vi "Dialog-Super Password.vi"(8 "error in":errorcluster, 11 "Please Enter the Developer Password":string) -> (0 "error out":errorcluster, 2 "Password Out":string, 3 "Cancelled?":bool)   [LabVIEW 2018]
doc: "Use this template to create a dialog box with event handling."
panel:
  in  "Yes":bool
  in  "Cancel":bool
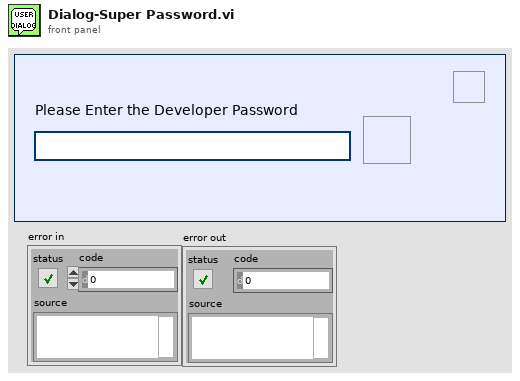
[diagram p1: front panel]
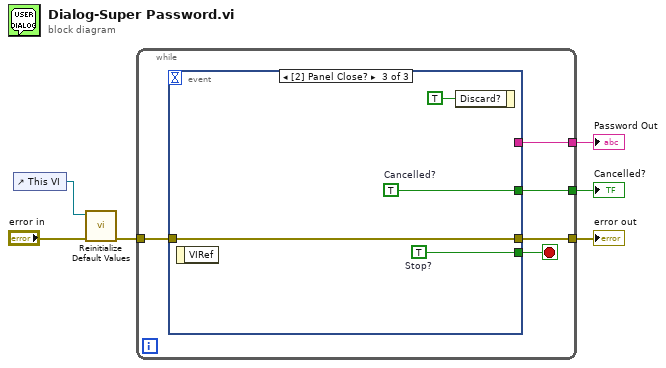
[diagram p0: block diagram]
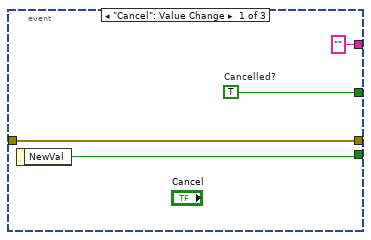
[diagram p2: hidden frame]
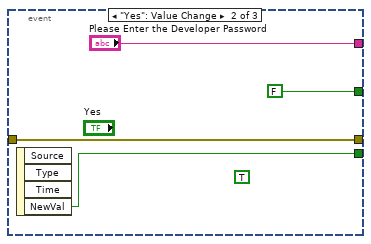
[diagram p3: hidden frame]
diagram:
  n1 = control-ref of="This VI"() -> (w1:refnum<vi>)
  n2 = call "Reinitialize Default Values.vi"("error in (no error)"="error in", "VI in"=w1) -> ("error out"=w2:errorcluster)  [unwired: 9 in]
  n3 = while {
    tunnel: [w10] -> w6
    tunnel: [w9] -> w5
    tunnel: w2 -> [w8]
    tunnel: [w7] -> w3
    stop <- w11 stop-if-true
    n4 = event shown="[2] Panel Close?" {
      selector: _ -> [_ _ _]
      dyn-events: _ -> [_ _ _]
      timeout: _ -> [_ _ _]
      tunnel: [w12 w16 w22] -> w11
      tunnel: [w15 FALSE w21] -> w10
      tunnel: ["" ("Please Enter the Developer Password") "Please Enter the Developer Password" _] -> w9
      tunnel: w8 -> [w14 w17 w20]
      tunnel: [w14 w17 w20] -> w7
      event "Cancel": Value Change {
        w15 = TRUE  # Cancelled?
        n5 = event-data() -> ("NewVal"=w12:bool)  [unwired: 1 in]
      }
      event "Yes": Value Change {
        (unwired) TRUE ("Stop?")
        n6 = event-data() -> ("NewVal"=w16:bool)  [unwired: 1 in, 3 out]
      }
      event Panel Close? {
        w21 = TRUE  # Cancelled?
        w22 = TRUE  # Stop?
        n7 = event-data() -> ()  [unwired: 1 in, 1 out]
        n8 = event-data("Discard?"=TRUE) -> ()  [unwired: 1 in, 1 out]
      }
    }
  }
  "Cancelled?" <- w6
  "Password Out" <- w5
  "error out" <- w3
